vi "Read Subscriber List.vi"(11 "Topic in":refnum<class "Topic.lvclass">) -> (0 "error out":errorcluster, 2 "Subscriber List":refnum<class "SubscriptionRequest.lvclass">[](array[class]))   [LabVIEW 2015, in "Mediator.lvlib" / "Topic.lvclass"]
uses:
  Topic.lvclass
  IMediator/SubscriptionRequest/SubscriptionRequest.lvclass
  Topic.lvclass/Topic.ctl
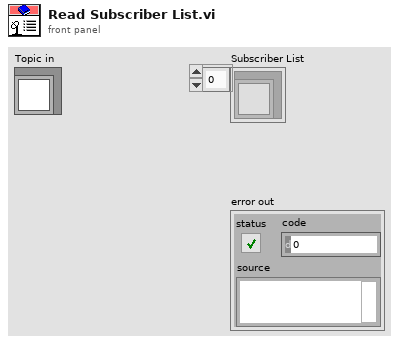
[diagram p1: front panel]
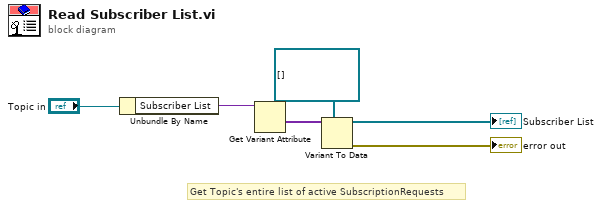
[diagram p0: block diagram]
diagram:
  # "Get Topic's entire list of active SubscriptionRequests"
  n1 = Unbundle By Name("Topic in") -> ("Subscriber List"=w6:variant)
  n2 = Get Variant Attribute(Variant=w6) -> (values=w1:variant[])  [unwired: 3 in, 3 out]
  n3 = Variant To Data(type=refnum<class "SubscriptionRequest.lvclass">[] [] ("Topic Enqueuer"), Variant=w1) -> (data=→"Subscriber List":refnum<class "SubscriptionRequest.lvclass">[], error out=→"error out":errorcluster)  [unwired: 1 in]
